vi "GetExplicitMessage_lowlevel.vi"(7 "Attribute":i32, 8 "error in (no error)":errorcluster, 9 "assembly instance ID":u32, 10 "Class":i32, 11 ".NET Refnum in":refnum<k24>) -> (0 "error out":errorcluster, 1 "GetAttributeSingle":u8[](array[numeric]), 2 "Numeric":i32, 3 ".NET Refnum out":refnum<k24>)   [LabVIEW 2022 SP3]
uses:
  C:/projects/Digilens_IPLC2/Classes/Motor Controller/EEIP.dll
  EEIP.dll
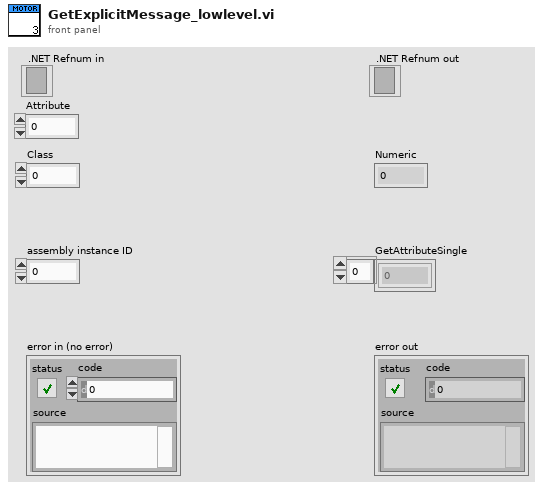
[diagram p1: front panel]
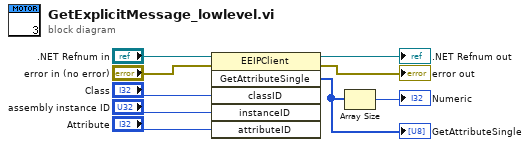
[diagram p0: block diagram]
diagram:
  n1 = invoke class="EEIPClient" method="GetAttributeSingle"(reference=".NET Refnum in", error in="error in (no error)", "classID"="Class", "instanceID"="assembly instance ID", "attributeID"="Attribute") -> (reference out=→".NET Refnum out":refnum<k24>, error out=→"error out":errorcluster, "GetAttributeSingle"=w5:u8[])  [unwired: 1 in, 3 out]
  "GetAttributeSingle" <- w5
  n2 = Array Size(array=w5) -> (size(s)=→"Numeric":i32)
